vi "DeInit.vi"(8 "error in (no error)":errorcluster, 11 "BPC30x in":refnum<class "BPC30x.lvclass">) -> (0 "error out":errorcluster, 3 "BPC30x out":refnum<class "BPC30x.lvclass">)   [LabVIEW 2023, in "TranslationStage Library.lvlib" / "BPC30x.lvlib" / "BPC30x.lvclass"]
uses:
  BPC30x.lvclass
  C:/Program Files/National Instruments/LabVIEW 2023/vi.lib/ActorFramework/Actor/Actor.lvclass
  BPC30x.lvclass/BPC30x.ctl
  <vilib>/ActorFramework/Actor/Actor.lvclass/Actor.ctl
  Interfaces/InitDeinitInterface/InitDeinitComm Messages/DeInit Done Msg/DeInit Done Msg.lvclass/DeInit Done Msg.ctl
  <vilib>/ActorFramework/Message Enqueuer/Message Enqueuer.lvclass/Message Enqueuer.ctl
  <vilib>/ActorFramework/Message Enqueuer/Enqueue.vi
  Interfaces/InitDeinitInterface/InitDeinitComm Messages/DeInit Done Msg/DeInit Done Msg.lvclass
  C:/Program Files/National Instruments/LabVIEW 2023/vi.lib/ActorFramework/Message/Message.lvclass
  <vilib>/ActorFramework/Message Priority Queue/Priority Enqueue.vi
  <vilib>/ActorFramework/Actor/Actor.lvclass
  C:/Users/quantum/Documents/LVDAQ/ConcreteClasses/ConcreteInstrumentClasses/BPC301/BPC30x/BPC30x.lvclass
  C:/Users/quantum/Documents/LVDAQ/Interfaces/InitDeinitInterface/InitDeinit/InitDeinit.lvclass
  C:/Users/quantum/Documents/LVDAQ/Interfaces/AbstractInstrumentClasses/TranslationStages_LV/TranslationStageInterface/TranslationStagesInterface.lvclass
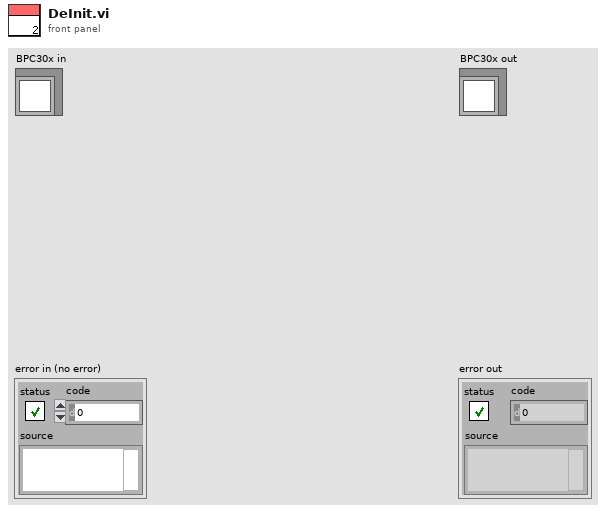
[diagram p1: front panel]
types:
  T1 = typedef "typedefs.lvlib/InstrumentData.ctl" = cluster{"Instr Error":errorcluster, "Address":cluster{"address type":enum16{"VISA", "Index"}, "Address":string, "instrument type":T2}, "CurrentState":cluster{"Initialized":bool, "Connected":bool, "Running":bool, "Error":bool}}
  T2 = typedef "typedefs.lvlib/instrumentType.ctl" = enum16{"Spectrometer", "Camera", "Stepper", "Piezo", "SLM"}
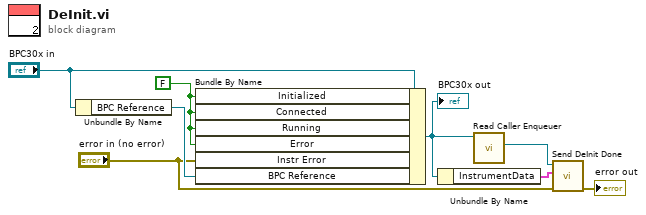
[diagram p0: block diagram]
diagram:
  w6 = FALSE ("InstrumentData.CurrentState.Connected")
  n1 = Unbundle By Name("BPC30x in") -> ("BPC Reference"=w7:refnum<k24>)
  n2 = Bundle By Name(cluster="BPC30x in", "Initialized"=w6, "Connected"=w6, "Running"=w6, "Error"=w6, "Instr Error"="error in (no error)", "BPC Reference"=w7) -> (w3:refnum<class "BPC30x.lvclass">)
  "BPC30x out" <- w3
  n3 = Unbundle By Name(w3) -> ("InstrumentData"=w2:T1)
  n4 = call <vilib>:"Read Caller Enqueuer.vi"("Actor"=w3) -> ("Caller Enqueuer"=w4:refnum<class "Message Enqueuer.lvclass">)  [unwired: 10 in]
  n5 = call "Send DeInit Done.vi"("error in (no error)"="error in (no error)", "InstrumentData"=w2, "Message Enqueuer"=w4) -> ("error out"=→"error out":errorcluster)  [unwired: 7 in, 1 out]
